vi "Reposition.vi"(11 "Cluster":T1) -> (3 "Cluster Out":T1)   [LabVIEW 2019, in "LSS.lvlib"]
doc: "Repositions front panel objects of example using property nodes.\n\n<b>Inputs:</b>\n<b>Cluster</b> - Cluster of front panel controls that will have style applied to them."
uses:
  LSS.lvlib
  Before UI References.ctl
  <vilib>/Utility/miscctls.llb/LVBoundsTypeDef.ctl
  <vilib>/Utility/miscctls.llb/LVPositionTypeDef.ctl
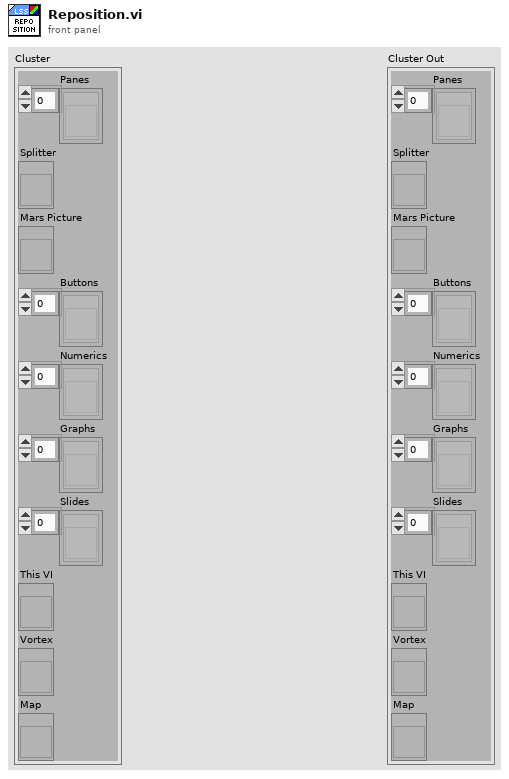
[diagram p1: front panel]
types:
  T1 = typedef "LSS.lvlib/Before UI References.ctl" = cluster{"Panes":refnum<vi>[], "Splitter":refnum<vi>, "Mars Picture":refnum<vi>, "Buttons":refnum<vi>[], "Numerics":refnum<vi>[], "Graphs":refnum<vi>[], "Slides":refnum<vi>[], "This VI":refnum<vi>, "Vortex":refnum<vi>, "Map":refnum<vi>}
  T2 = typedef "LVBoundsTypeDef.ctl" = cluster{"Width":u32, "Height":u32}
  T3 = typedef "LVPositionTypeDef.ctl" = cluster{"Left":i32, "Top":i32}
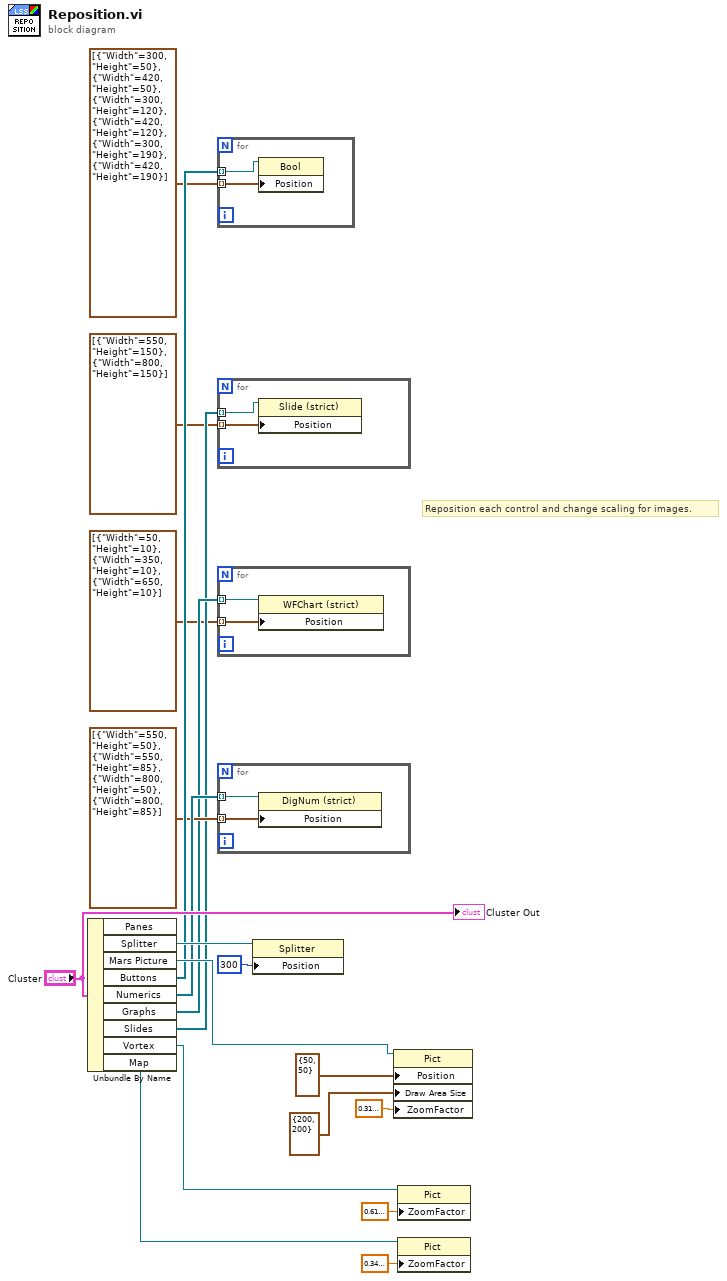
[diagram p0: block diagram]
diagram:
  # "Reposition each control and change scaling for images."
  n1 = Unbundle By Name("Cluster") -> ("Splitter"=w18:refnum<vi>, "Mars Picture"=w19:refnum<vi>, "Buttons"=w14:refnum<vi>[], "Numerics"=w12:refnum<vi>[], "Graphs"=w10:refnum<vi>[], "Slides"=w9:refnum<vi>[], "Vortex"=w4:refnum<vi>, "Map"=w3:refnum<vi>)  [unwired: 1 out]
  n2 = for {
    tunnel: w14 -> [w21] mode=indexing
    tunnel: T2[] [{"Width"=300, "Height"=50}, {"Width"=420, "Height"=50}, {"Width"=300, "Height"=120}, {"Width"=420, "Height"=120}, {"Width"=300, "Height"=190}, {"Width"=420, "Height"=190}] ("Button Size") -> [w20] mode=indexing
    n3 = property on="Property Node" class="Bool"(reference=w21, "Position"=w20) -> ()  [unwired: 1 in, 2 out]
  }
  n4 = for {
    tunnel: w9 -> [w23] mode=indexing
    tunnel: T2[] [{"Width"=550, "Height"=150}, {"Width"=800, "Height"=150}] ("Button Size") -> [w22] mode=indexing
    n5 = property class="Slide (strict)"(reference=w23, "Position"=w22) -> ()  [unwired: 1 in, 2 out]
  }
  n6 = for {
    tunnel: w10 -> [w25] mode=indexing
    tunnel: T2[] [{"Width"=50, "Height"=10}, {"Width"=350, "Height"=10}, {"Width"=650, "Height"=10}] ("Button Size") -> [w24] mode=indexing
    n7 = property class="WFChart (strict)"(reference=w25, "Position"=w24) -> ()  [unwired: 1 in, 2 out]
  }
  n8 = for {
    tunnel: w12 -> [w27] mode=indexing
    tunnel: T2[] [{"Width"=550, "Height"=50}, {"Width"=550, "Height"=85}, {"Width"=800, "Height"=50}, {"Width"=800, "Height"=85}] ("Button Size") -> [w26] mode=indexing
    n9 = property class="DigNum (strict)"(reference=w27, "Position"=w26) -> ()  [unwired: 1 in, 2 out]
  }
  n10 = property on="Property Node" class="Splitter"(reference=w18, "Position"=300 ("Splitter Position")) -> ()  [unwired: 1 in, 2 out]
  n11 = property on="Property Node" class="Pict"(reference=w19, "Position"=T3 {"Left"=50, "Top"=50}, "Draw Area Size"=T2 {"Width"=200, "Height"=200}, "ZoomFactor"=sgl 0.32 ("Zoom Factor")) -> ()  [unwired: 1 in, 2 out]
  n12 = property on="Property Node" class="Pict"(reference=w4, "ZoomFactor"=sgl 0.61 ("Zoom Factor")) -> ()  [unwired: 1 in, 2 out]
  n13 = property on="Property Node" class="Pict"(reference=w3, "ZoomFactor"=sgl 0.35 ("Zoom Factor")) -> ()  [unwired: 1 in, 2 out]
  "Cluster Out" <- "Cluster"
